vi "_19_Sample_qsns_06[22].vi"() -> ()   [LabVIEW 2020]
panel:
  out "subarray":i32[](array[numeric])
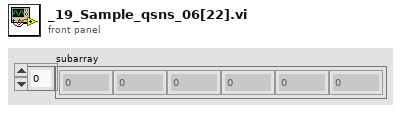
[diagram p1: front panel]
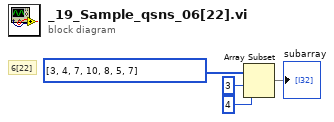
[diagram p0: block diagram]
diagram:
  # "6[22]"
  n1 = Array Subset(array=i32[] [3, 4, 7, 10, 8, 5, 7], index=3, length=4) -> (→"subarray":i32[])
